vi "Convert plane for terastitcher.vi"(0 "Image in":T1, 1 "File Handle":u32, 2 "downcast to 8-bit? (F)":bool, 3 "z start position":i32, 5 "file in":path, 9 "Frame Index":i32=-1, 11 "error in (no error)":errorcluster, 12 "basepath name":string, 14 "z step size":i32) -> (4 "Image out":T1, 15 "error out":errorcluster)   [LabVIEW 2012]
uses:
  <vilib>/vision/Image Controls.llb/IMAQ Image.ctl
  <vilib>/vision/NI_Vision_Development_Module.lvlib
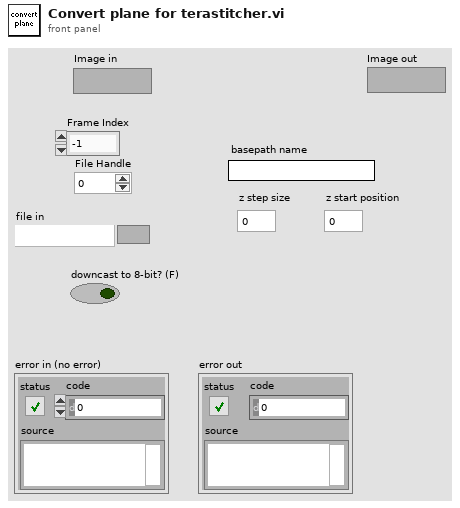
[diagram p1: front panel]
types:
  T1 = typedef "IMAQ Image.ctl" = refnum<image>
  T2 = cluster{"Rows Per Strip":i32, "Photometric":i32, "Compression Type":i32}
  T3 = typedef "Image Type" = u32
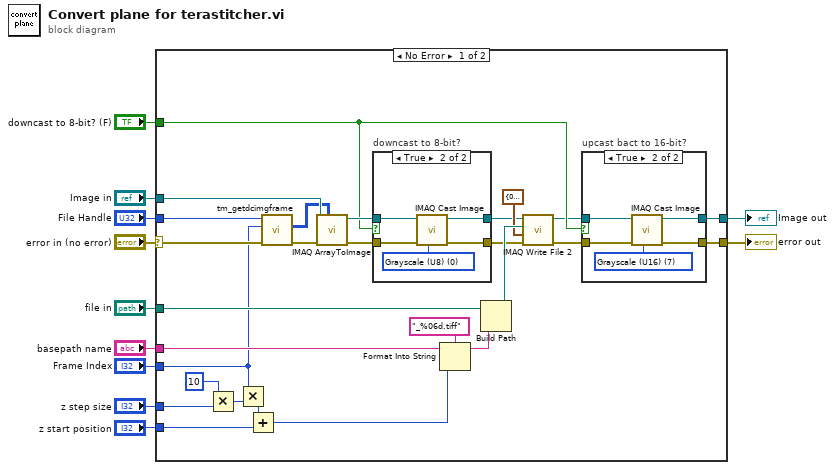
[diagram p0: block diagram]
diagram:
  n1 = case shown="No Error" "error in (no error)" {
    selector: "error in (no error)" -> [w36 w54]
    tunnel: "File Handle" -> [w38 _]
    tunnel: "file in" -> [w32 _]
    tunnel: [w14 w54] -> w9
    tunnel: "Frame Index" -> [w27 _]
    tunnel: "Image in" -> [w35 w53]
    tunnel: [w12 w53] -> w6
    tunnel: "basepath name" -> [w28 _]
    tunnel: "z step size" -> [w22 _]
    tunnel: "z start position" -> [w25 _]
    tunnel: "downcast to 8-bit? (F)" -> [w16 _]
    frame No Error {
      n2 = Multiply(x=10 ("y"), y=w22) -> (x*y=w21:i32)
      n3 = Multiply(x=w27, y=w21) -> (x*y=w26:i32)
      n4 = Add(x=w26, y=w25) -> (x+y=w24:i32)
      n5 = call <userlib>:"tm_getdcimgframe.vi"("error in (no error)"=w36, "Frame Index"=w27, "File Handle in"=w38) -> ("error out"=w30:errorcluster, "Data"=w31:u16[][])  [unwired: 5 in, 2 out]
      n6 = call "IMAQ ArrayToImage"("Image Pixels (U16)"=w31, "error in (no error)"=w30, "Image"=w35) -> ("error out"=w19:errorcluster, "Image Out"=w20:T1)  [unwired: 7 in]
      n7 = case "downcast to 8-bit?" shown="True" w16 {
        tunnel: w20 -> [w46 w50]
        tunnel: w19 -> [w47 w48]
        tunnel: [w47 w52] -> w18
        tunnel: [w46 w49] -> w17
        frame False {
        }
        frame True {
          w51 = T3 0 items=["Grayscale (U8)", "Grayscale (I16)", "Grayscale (SGL)", "Complex (CSG)", "RGB (U32)", "HSL (U32)", "RGB (U64)", "Grayscale (U16)"] ("Image Type")
          n8 = call "IMAQ Cast Image"("Image Type"=w51, "error in (no error)"=w48, "Image Src"=w50) -> ("error out"=w52:errorcluster, "Image Dst Out"=w49:T1)  [unwired: 7 in]
        }
      }
      n9 = Format Into String(format string="_%06d.tiff", initial string=w28, w24) -> (resulting string=w33:string)  [unwired: 1 in, 1 out]
      n10 = Build Path(base path=w32, name or relative path=w33) -> (appended path=w37:path)
      n11 = call-poly "IMAQ Write File 2"("error in (no error)"=w18, "TIFF Options"=T2 {"Rows Per Strip"=0, "Photometric"=1, "Compression Type"=0}, "File Path"=w37, "Image"=w17) -> ("error out"=w15:errorcluster, "Image Out (duplicate)"=w13:T1)  [unwired: 6 in]
      n12 = case "upcast bact to 16-bit?" shown="True" w16 {
        tunnel: w13 -> [w39 w43]
        tunnel: w15 -> [w40 w41]
        tunnel: [w40 w45] -> w14
        tunnel: [w39 w42] -> w12
        frame False {
        }
        frame True {
          w44 = T3 7 items=["Grayscale (U8)", "Grayscale (I16)", "Grayscale (SGL)", "Complex (CSG)", "RGB (U32)", "HSL (U32)", "RGB (U64)", "Grayscale (U16)"] ("Image Type")
          n13 = call "IMAQ Cast Image"("Image Type"=w44, "error in (no error)"=w41, "Image Src"=w43) -> ("error out"=w45:errorcluster, "Image Dst Out"=w42:T1)  [unwired: 7 in]
        }
      }
    }
    frame Error {
    }
  }
  "error out" <- w9
  "Image out" <- w6
